vi "GetDescriptionNodeText.vi"(8 "Error In":errorcluster, 11 "Pattern Node In":refnum<k20>) -> (0 "Error Out":errorcluster, 2 "Description":string, 3 "Pattern Node Out":refnum<k20>)   [LabVIEW 2012, in "Virtual-PGA.lvlib"]
uses:
  Virtual-PGA.lvlib
  <vilib>/xml/NI_XML.lvlib
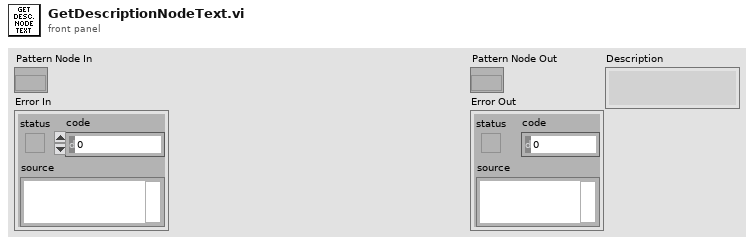
[diagram p1: front panel]
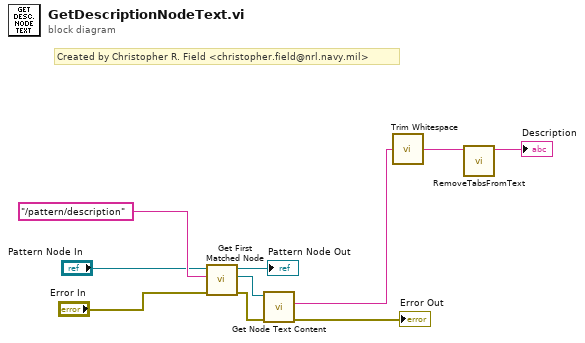
[diagram p0: block diagram]
diagram:
  # "Created by Christopher R. Field <christopher.field@nrl.navy.mil>"
  n1 = call <vilib>:"Get First Matched Node.vi"("error in (no error)"="Error In", "XPath expression"="/pattern/description", "node in"="Pattern Node In") -> ("error out"=w8:errorcluster, "node result"=w9:refnum<k20>, "node out"=→"Pattern Node Out":refnum<k20>)  [unwired: 6 in]
  n2 = call <vilib>:"Get Node Text Content.vi"("error in (no error)"=w8, "node in"=w9) -> ("error out"=→"Error Out":errorcluster, "node text"=w2:string)  [unwired: 7 in, 1 out]
  n3 = call <vilib>:"Trim Whitespace.vi"("string"=w2) -> ("trimmed string"=w3:string)  [unwired: 1 in]
  n4 = call "RemoveTabsFromText.vi"("Tabbed Text"=w3) -> ("Non-Tabbed Text"=→"Description":string)  [unwired: 10 in]
